vi "enable debugging.vi"() -> ()   [LabVIEW 2013]
panel:
  out "error out":errorcluster
  in  "Folder Path":path
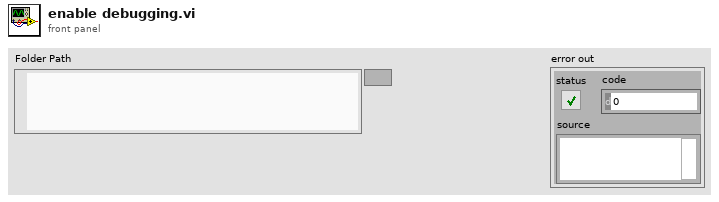
[diagram p1: front panel]
types:
  T1 = enum32{"Bad", "Idle", "Run top level", "Running"}
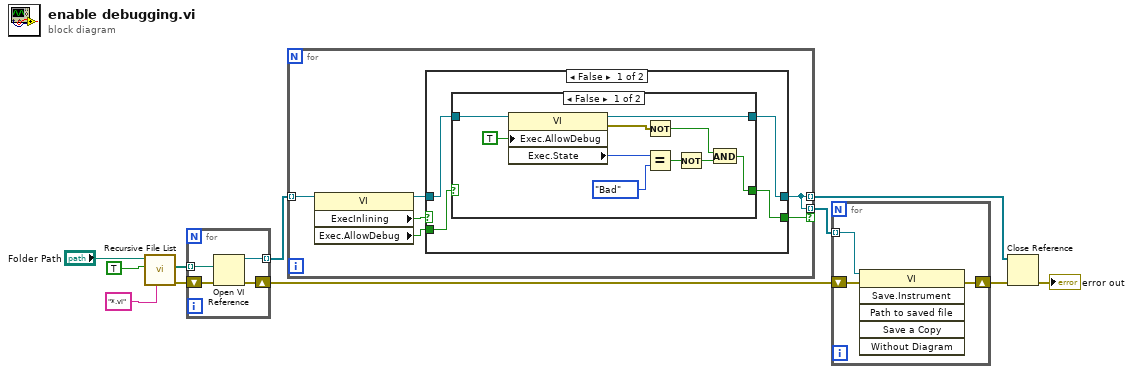
[diagram p0: block diagram]
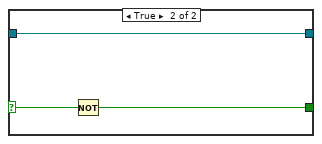
[diagram p2: hidden frame]
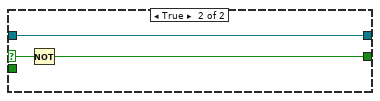
[diagram p3: hidden frame]
diagram:
  n1 = call <vilib>:"Recursive File List.vi"("pattern"="*.vi", "Treat LLBs as Folders?"=TRUE, "Folder Path"="Folder Path") -> ("error out"=w3:errorcluster, "All Files in Dir"=w8:path[])  [unwired: 4 in, 3 out]
  n2 = for {
    tunnel: w8 -> [w15] mode=indexing
    tunnel: [w14] -> w7 mode=indexing
    shift-right: [w13] -> w4
    shift-left: w3 -> [w12]
    n3 = Open VI Reference(vi path=w15, error in (no error)=w12) -> (vi reference=w14:refnum<vi>, error out=w13:errorcluster)  [unwired: 4 in]
  }
  n4 = for {
    tunnel: w7 -> [w21] mode=indexing
    tunnel: [w18] -> w6 mode=indexing
    tunnel: [w18] -> w1 mode=indexing if=w17
    n5 = property class="VI"(reference=w21) -> (reference out=w20:refnum<vi>, "ExecInlining"=w19:bool, "Exec.AllowDebug"=w16:bool)  [unwired: 1 in, 1 out]
    n6 = case shown="False" w19 {
      selector: w19 -> [_ w40]
      tunnel: w20 -> [w25 w41]
      tunnel: [w22 w41] -> w18
      tunnel: [w23 w39] -> w17
      tunnel: w16 -> [w24 _]
      frame False {
        n7 = case shown="False" w24 {
          selector: w24 -> [_ w38]
          tunnel: w25 -> [w33 w36]
          tunnel: [w28 w37] -> w23
          tunnel: [w32 w36] -> w22
          frame False {
            n8 = property class="VI"(reference=w33, "Exec.AllowDebug"=TRUE ("Execution:Allow Debugging")) -> (reference out=w32:refnum<vi>, error out=w34:errorcluster, "Exec.State"=w30:T1)  [unwired: 1 in]
            n9 = Not(x=w34) -> (.not. x?=w35:bool)
            n10 = Equal?(x=w30, y=T1."Bad") -> (x = y?=w26:bool)
            n11 = Not(x=w26) -> (.not. x?=w27:bool)
            n12 = And(x=w35, y=w27) -> (x .and. y?=w28:bool)
          }
          frame True {
            n13 = Not(x=w38) -> (.not. x?=w37:bool)
          }
        }
      }
      frame True {
        n14 = Not(x=w40) -> (.not. x?=w39:bool)
      }
    }
  }
  n15 = for {
    shift-right: [w44] -> w5
    shift-left: w4 -> [w43]
    tunnel: w1 -> [w42] mode=indexing
    n16 = invoke class="VI" method="Save.Instrument"(reference=w42, error in=w43) -> (error out=w44:errorcluster)  [unwired: 4 in, 5 out]
  }
  n17 = Close Reference(reference=w6, error in (no error)=w5) -> (error out=→"error out":errorcluster)
